vi "signal_log.vi"(8 "error in":errorcluster, 9 "Demodulated signals":waveform(dbl)[][](array[waveform]), 11 "Log file refnum":refnum<file>) -> (0 "error out":errorcluster)   [LabVIEW 2010]
uses:
  <vilib>/Waveform/WDTOps.llb/WDT Get Waveform Time Array DBL.vi
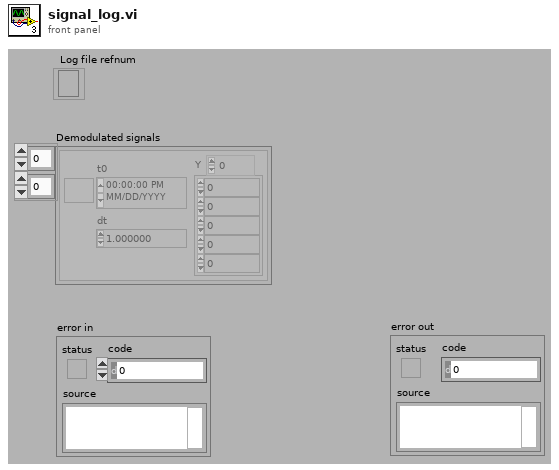
[diagram p1: front panel]
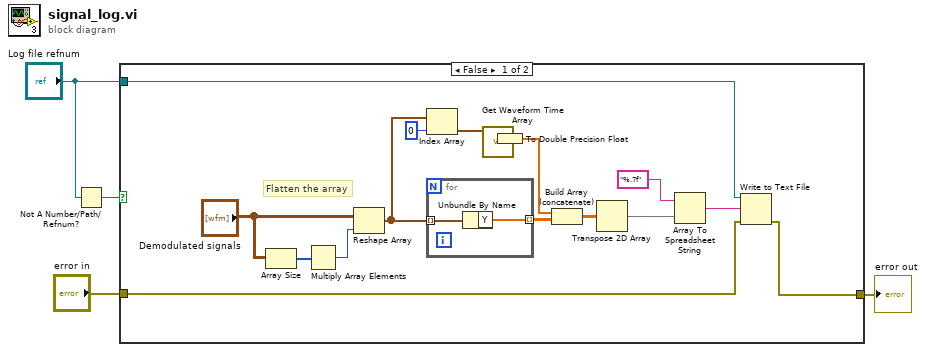
[diagram p0: block diagram]
diagram:
  n1 = Not A Number/Path/Refnum?(number/path/refnum="Log file refnum") -> (NaN/Path/Refnum?=w4:bool)
  n2 = case shown="False" w4 {
    tunnel: "Log file refnum" -> [w9 _]
    tunnel: "error in" -> [w7 w23]
    tunnel: [w6 w23] -> w1
    frame False {
      # "Flatten the array"
      n3 = Array Size(array="Demodulated signals") -> (size(s)=w19:i32[])
      n4 = Multiply Array Elements(1:w19) -> (0:w20:i32)
      n5 = Reshape Array("Demodulated signals", w20) -> (w16:waveform(dbl)[])
      n6 = Index Array(array=w16, index=0) -> (element=w14:waveform(dbl))
      n7 = for {
        tunnel: w16 -> [w22] mode=indexing
        tunnel: [w21] -> w17 mode=indexing
        n8 = Unbundle By Name(w22) -> ("Y"=w21:dbl[])
      }
      n9 = call-poly <vilib>:"Get Waveform Time Array.vi"("waveform in"=w14) -> ("X array"=w5:timestamp[])  [unwired: 1 in, 9 out]
      n10 = To Double Precision Float(number=w5) -> (double precision float=w13:dbl[])
      n11 = Build Array (concatenate)(w13, w17) -> (w11:dbl[][])
      n12 = Transpose 2D Array(2D array=w11) -> (transposed array=w10:dbl[][])
      n13 = Array To Spreadsheet String(array=w10, 3:"%.7f" ("format (%.3f)")) -> (spreadsheet string=w8:string)  [unwired: 1 out]
      n14 = Write to Text File(file (use dialog)=w9, text=w8, error in=w7) -> (error out=w6:errorcluster)  [unwired: 3 out]
    }
    frame True {
    }
  }
  "error out" <- w1
